vi "Create PB Response.vi"(8 "error in (no error)":errorcluster, 10 "Protobuf Message":refnum<class "Message.lvclass">, 11 "Status Code":u16) -> (0 "error out":errorcluster, 3 "ProtobufResponse out":refnum<class "ProtobufResponse.lvclass">)   [LabVIEW 2020, in "ProtobufResponse.lvclass"]
uses:
  ProtobufResponse.lvclass
  ProtobufResponse.lvclass/ProtobufResponse.ctl
  lv-http-util/HTTP Utils/Response/Response.lvclass
  lv-protoc/LV-Proto/Message/Message.lvclass
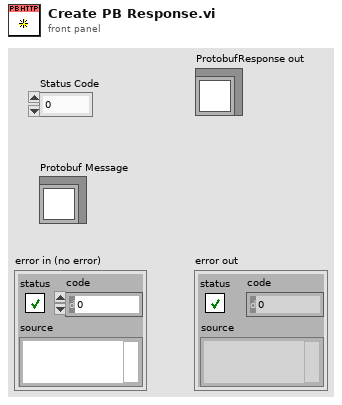
[diagram p1: front panel]
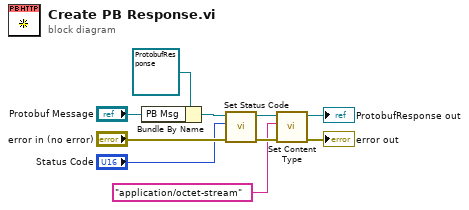
[diagram p0: block diagram]
diagram:
  n1 = Bundle By Name(cluster=refnum<class "ProtobufResponse.lvclass"> refnum ("ProtobufResponse in"), "PB Msg"="Protobuf Message") -> (w8:refnum<class "ProtobufResponse.lvclass">)
  n2 = call "Set Status Code.vi"("error in (no error)"="error in (no error)", "Status Code"="Status Code", "Response in"=w8) -> ("error out"=w4:errorcluster, "Response out"=w5:refnum<class "ProtobufResponse.lvclass">)  [unwired: 7 in]
  n3 = call "Set Content Type.vi"("error in (no error)"=w4, "Content-Type"="application/octet-stream", "Response in"=w5) -> ("error out"=→"error out":errorcluster, "Response out"=→"ProtobufResponse out":refnum<class "ProtobufResponse.lvclass">)  [unwired: 7 in]
